vi "Analysis.Generate First and Last Pass Result Summaries form 2D Data.vi"(10 "Data":string[][](array[string]), 11 "Header":string[](array[string])) -> (1 "Lists":T1, 3 "ResultSum":T2[](array[typedef]))   [LabVIEW 2024]
uses:
  Analysis.Result Summary.ctl
  Analysis.Result Summary Lists.ctl
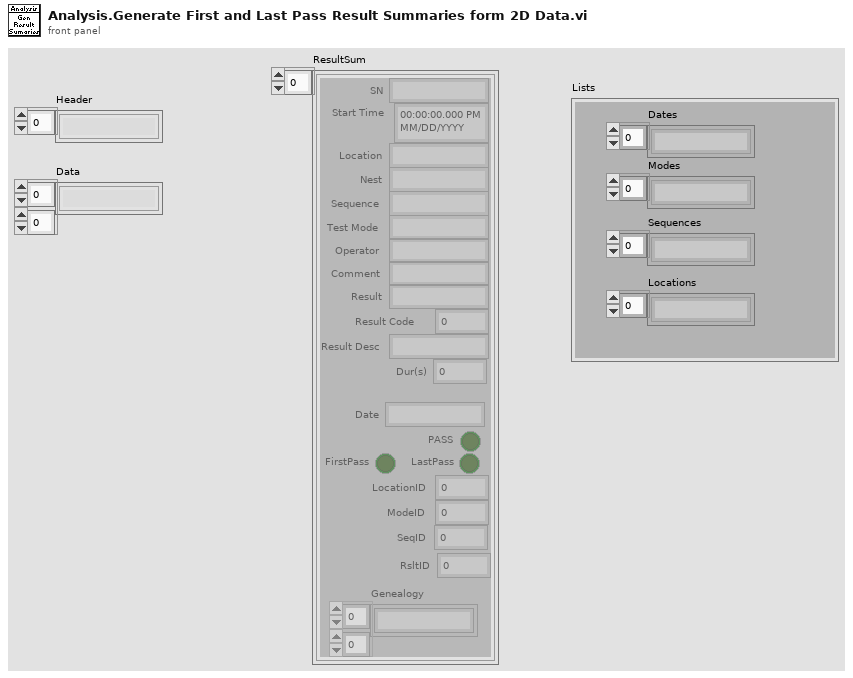
[diagram p1: front panel]
types:
  T1 = typedef "Analysis.Result Summary Lists.ctl" = cluster{"Dates":string[], "Modes":string[], "Sequences":string[], "Locations":string[]}
  T2 = typedef "Analysis.Result Summary.ctl" = cluster{"SN":string, "Start Time":timestamp, "Location":string, "Nest":string, "Sequence":string, "Operator":string, "Test Mode":string, "Comment":string, "Result":string, "Result Code":i32, "Result Desc":string, "Date":string, "Dur(s)":dbl, "PASS":bool, "FirstPass":bool, "LastPass":bool, "LocationID":i32, "ModeID":i32, "SeqID":i32, "RsltID":i32, "Genealogy":string[][]}
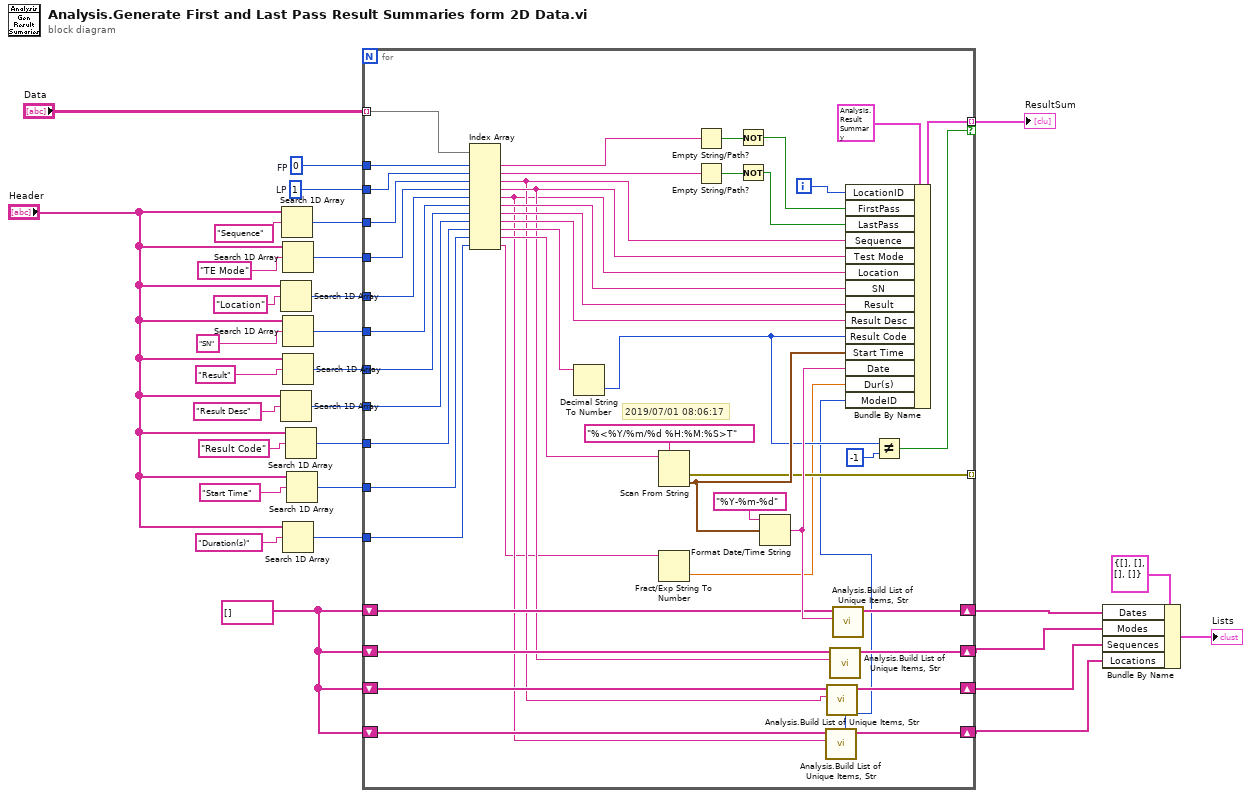
[diagram p0: block diagram]
diagram:
  w10 = string[] []
  w26 = 1  # LP
  w27 = 0  # FP
  n1 = Search 1D Array(1D array="Header", element="Location") -> (index of element=w23:i32)  [unwired: 1 in]
  n2 = Search 1D Array(1D array="Header", element="Result Desc") -> (index of element=w17:i32)  [unwired: 1 in]
  n3 = Search 1D Array(1D array="Header", element="Sequence") -> (index of element=w25:i32)  [unwired: 1 in]
  n4 = Search 1D Array(1D array="Header", element="TE Mode") -> (index of element=w24:i32)  [unwired: 1 in]
  n5 = Search 1D Array(1D array="Header", element="SN") -> (index of element=w20:i32)  [unwired: 1 in]
  n6 = Search 1D Array(1D array="Header", element="Result") -> (index of element=w19:i32)  [unwired: 1 in]
  n7 = Search 1D Array(1D array="Header", element="Duration(s)") -> (index of element=w1:i32)  [unwired: 1 in]
  n8 = Search 1D Array(1D array="Header", element="Result Code") -> (index of element=w14:i32)  [unwired: 1 in]
  n9 = Search 1D Array(1D array="Header", element="Start Time") -> (index of element=w13:i32)  [unwired: 1 in]
  n10 = for {
    tunnel: "Data" -> [w77] mode=indexing
    tunnel: w27 -> [w78]
    tunnel: w26 -> [w76]
    tunnel: w25 -> [w75]
    tunnel: w24 -> [w74]
    tunnel: w23 -> [w73]
    tunnel: w20 -> [w70]
    tunnel: w19 -> [w69]
    tunnel: [w56] -> w11 mode=indexing if=w36
    tunnel: w17 -> [w65]
    tunnel: w14 -> [w64]
    tunnel: w13 -> [w63]
    shift-right: [w51] -> w9
    shift-left: w10 -> [w52]
    shift-right: [w50] -> w8
    shift-left: w10 -> [w49]
    shift-right: [w47] -> w7
    shift-left: w10 -> [w48]
    shift-right: [w45] -> w6
    shift-left: w10 -> [w44]
    tunnel: [w39] -> _ mode=indexing
    tunnel: w1 -> [w35]
    i -> [w32]
    # "2019/07/01 08:06:17"
    n11 = Index Array(array=w77, index #1=w78, index #2=w76, index #3=w75, index #4=w74, index #5=w73, index #6=w70, index #7=w69, index #8=w65, index #9=w64, index #10=w63, index #11=w35) -> (element #1=w72:string, element #2=w71:string, element #3=w43:string, element #4=w46:string, element #5=w42:string, element #6=w61:string, element #7=w60:string, element #8=w59:string, element #9=w58:string, element #10=w57:string, element #11=w33:string)
    n12 = Decimal String To Number(string=w58) -> (number=w37:i32)  [unwired: 2 in, 1 out]
    n13 = Scan From String(format string="%<%Y/%m/%d %H:%M:%S>T", input string=w57) -> (error out=w39:errorcluster, output 1=w55:timestamp)  [unwired: 3 in, 2 out]
    n14 = Fract/Exp String To Number(string=w33) -> (number=w34:dbl)  [unwired: 3 in, 1 out]
    n15 = Empty String/Path?(string/path=w72) -> (empty?=w68:bool)
    n16 = Empty String/Path?(string/path=w71) -> (empty?=w67:bool)
    n17 = Not(x=w68) -> (.not. x?=w41:bool)
    n18 = Not(x=w67) -> (.not. x?=w40:bool)
    n19 = Format Date/Time String(time format string (%c)="%Y-%m-%d", seconds (now)=w55) -> (date/time string=w53:string)  [unwired: 1 in]
    n20 = call "Analysis.Build List of Unique Items, Str.vi"("Item In"=w42, "List In"=w44) -> ("List Out"=w45:string[], "Index"=w31:i32)  [unwired: 7 in, 1 out]
    n21 = call "Analysis.Build List of Unique Items, Str.vi"("Item In"=w43, "List In"=w48) -> ("List Out"=w47:string[])  [unwired: 7 in, 2 out]
    n22 = call "Analysis.Build List of Unique Items, Str.vi"("Item In"=w46, "List In"=w49) -> ("List Out"=w50:string[])  [unwired: 7 in, 2 out]
    n23 = call "Analysis.Build List of Unique Items, Str.vi"("Item In"=w53, "List In"=w52) -> ("List Out"=w51:string[])  [unwired: 7 in, 2 out]
    n24 = Bundle By Name(cluster=T2 {"SN"="", "Start Time"=timestamp(0 s since 1904-01-01), "Location"="", "Nest"="", "Sequence"="", "Operator"="", "Test Mode"="", "Comment"="", "Result"="", "Result Code"=0, "Result Desc"="", "Date"="", "Dur(s)"=0.0, "PASS"=FALSE, "FirstPass"=FALSE, "LastPass"=FALSE, "LocationID"=0, "ModeID"=0, "SeqID"=0, "RsltID"=0, "Genealogy"=[]} ("Result Summary"), "LocationID"=w32, "FirstPass"=w41, "LastPass"=w40, "Sequence"=w43, "Test Mode"=w46, "Location"=w42, "SN"=w61, "Result"=w60, "Result Desc"=w59, "Result Code"=w37, "Start Time"=w55, "Date"=w53, "Dur(s)"=w34, "ModeID"=w31) -> (w56:T2)
    n25 = Not Equal?(x=w37, y=-1) -> (x != y?=w36:bool)
  }
  "ResultSum" <- w11
  n26 = Bundle By Name(cluster=T1 {"Dates"=[], "Modes"=[], "Sequences"=[], "Locations"=[]} ("Lists"), "Dates"=w9, "Modes"=w8, "Sequences"=w7, "Locations"=w6) -> (→"Lists":T1)
